vi "KeyenceCVX.Main.ScanAck.vi"(4 "ReadImg":bool, 5 "Retries":i32, 6 "Timeout_ms":i32, 7 "TriggerNo":T1 items=["1"=1, "2"=2, "3"=3, "4"=4, "ALL"=5], 8 "error in (no error)":errorcluster, 9 "FTPPath":path, 10 "ImgPath":path, 11 "TCP Network Connection in":refnum<k5>) -> (0 "error out":errorcluster, 1 "ReadOut":string, 2 "ImgPathB":path, 3 "TCP Network Connection out":refnum<k5>)   [LabVIEW 2016]
uses:
  private/controls/TriggerNo.ctl
  Keyence/LowLevel/Keyence.Global.vi
  Station/Station.Global.vi
panel:
  out "ImgPathA":path
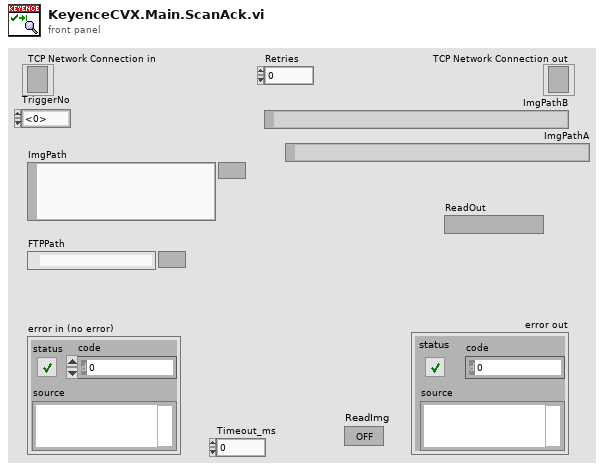
[diagram p1: front panel]
types:
  T1 = typedef "TriggerNo.ctl" = u8
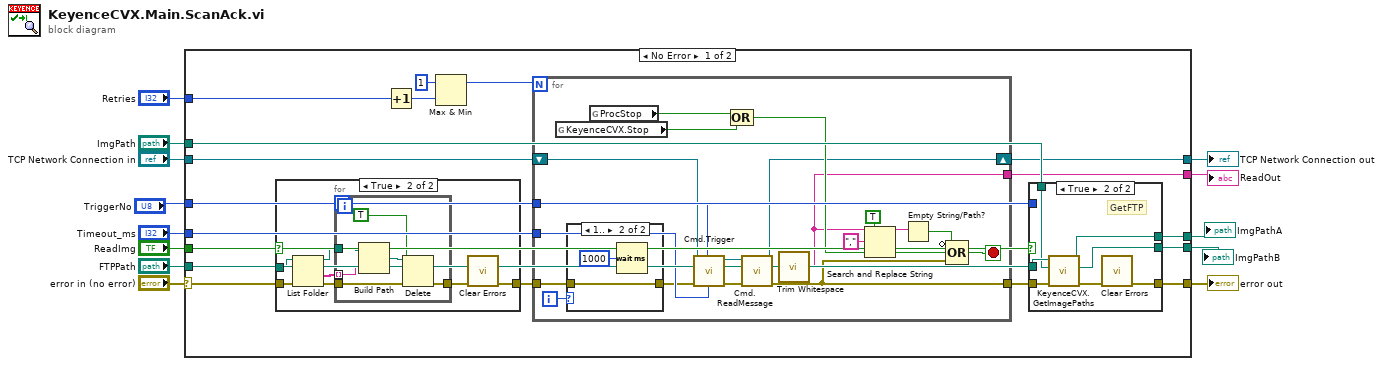
[diagram p0: block diagram]
diagram:
  n1 = case shown="No Error" "error in (no error)" {
    selector: "error in (no error)" -> [w17 w78]
    tunnel: "TriggerNo" -> [w31 _]
    tunnel: "ReadImg" -> [w30 _]
    tunnel: "FTPPath" -> [w14 _]
    tunnel: "ImgPath" -> [w29 _]
    tunnel: [w27 _] -> w10
    tunnel: [w26 w78] -> w9
    tunnel: "Timeout_ms" -> [w23 _]
    tunnel: "Retries" -> [w20 _]
    tunnel: [w19 w77] -> w6
    tunnel: "TCP Network Connection in" -> [w18 w77]
    tunnel: [w16 _] -> w2
    tunnel: [w15 _] -> w1
    frame No Error {
      n2 = case shown="True" w30 {
        tunnel: w17 -> [w32 w36]
        tunnel: [w32 w39] -> w28
        tunnel: w14 -> [_ w33]
        frame False {
        }
        frame True {
          n3 = List Folder(path=w33, error in=w36) -> (path out=w37:path, folder names=w38:string[], error out=w35:errorcluster)  [unwired: 2 in, 1 out]
          n4 = for {
            tunnel: w37 -> [w44]
            tunnel: w38 -> [w43] mode=indexing
            tunnel: w35 -> [w41]
            tunnel: [w40] -> w34
            n5 = Build Path(base path=w44, name or relative path=w43) -> (appended path=w42:path)
            n6 = Delete(path (use dialog)=w42, entire hierarchy (F)=TRUE, error in=w41) -> (error out=w40:errorcluster)  [unwired: 2 in, 2 out]
          }
          n7 = call <vilib>:"Clear Errors.vi"("error in (no error)"=w34) -> ("error out"=w39:errorcluster)  [unwired: 5 in, 1 out]
        }
      }
      n8 = Increment(x=w20) -> (x+1=w21:i32)
      n9 = Max & Min(x=1, y=w21) -> (max(x,y)=w24:i32)  [unwired: 1 out]
      n10 = for {
        N: w24 -> [_]
        shift-right: [w53] -> w19
        shift-left: w18 -> [w59]
        tunnel: w28 -> [w64]
        tunnel: [w52] -> w25
        tunnel: w31 -> [w58]
        tunnel: w23 -> [w57]
        tunnel: [w46] -> w27
        i -> [w63]
        stop <- w65 stop-if-true
        n11 = global read "Keyence.Global.vi" "KeyenceCVX.Stop"() -> (w61:bool)
        n12 = case shown="1.." w63 {
          tunnel: [w66 w68] -> w56
          tunnel: w64 -> [w66 w68]
          frame Default {
          }
          frame 1.. {
            n13 = Wait (ms)(milliseconds to wait=u32 1000) -> ()  [unwired: 1 out]
          }
        }
        n14 = global read "Station.Global.vi" "ProcStop"() -> (w62:bool)
        n15 = call "Cmd.Trigger.vi"("Timeout [ms] (1000)"=w57, "error in"=w56, "TriggerNo"=w58, "cID in"=w59) -> ("error out"=w55:errorcluster, "cID out"=w54:refnum<k5>)  [unwired: 5 in, 1 out]
        n16 = Compound Arithmetic op=OR(w62, w61) -> (w60:bool)
        n17 = call "Cmd.ReadMessage.vi"("error in"=w55, "cID in"=w54) -> ("error out"=w52:errorcluster, "Message"=w47:string, "cID out"=w53:refnum<k5>)  [unwired: 7 in]
        n18 = call <vilib>:"Trim Whitespace.vi"("string"=w47) -> ("trimmed string"=w46:string)  [unwired: 1 in]
        n19 = Search and Replace String(replace all?=TRUE ("replace all? (F)"), input string=w46, search string=",") -> (result string=w49:string)  [unwired: 5 in, 3 out]
        n20 = Empty String/Path?(string/path=w49) -> (empty?=w48:bool)
        n21 = Compound Arithmetic op=OR(invert w48, w60, w52) -> (w65:bool)
      }
      n22 = case shown="True" w30 {
        tunnel: w25 -> [w69 w75]
        tunnel: [w69 w76] -> w26
        tunnel: w29 -> [_ w70]
        tunnel: w31 -> [_ _]
        tunnel: [_ w73] -> w16
        tunnel: [_ w72] -> w15
        tunnel: w14 -> [_ w71]
        frame False {
        }
        frame True {
          # "GetFTP"
          n23 = call "KeyenceCVX.GetImagePaths.vi"("error in"=w75, "ImageFolder"=w70, "FTPPath"=w71) -> ("error out"=w74:errorcluster, "ImgPathB"=w72:path, "ImgPathA"=w73:path)  [unwired: 6 in]
          n24 = call <vilib>:"Clear Errors.vi"("error in (no error)"=w74) -> ("error out"=w76:errorcluster)  [unwired: 5 in, 1 out]
        }
      }
    }
    frame Error {
    }
  }
  "ImgPathB" <- w1
  "error out" <- w9
  "TCP Network Connection out" <- w6
  "ReadOut" <- w10
  "ImgPathA" <- w2
